vi "Read Current Paths.vi"(11 "PathControl in":refnum<class "PathControl.lvclass">) -> (2 "Current Paths":T1(array[cluster]), 3 "PathControl out":refnum<class "PathControl.lvclass">)   [LabVIEW 2020, in "PathControl.lvclass"]
uses:
  PathControl.lvclass
  PathControl.lvclass/PathControl.ctl
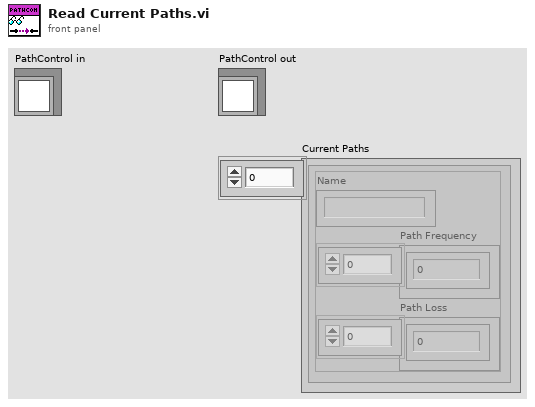
[diagram p1: front panel]
types:
  T1 = cluster{"Name":string, "Path Frequency":dbl[], "Path Loss":dbl[]}[]
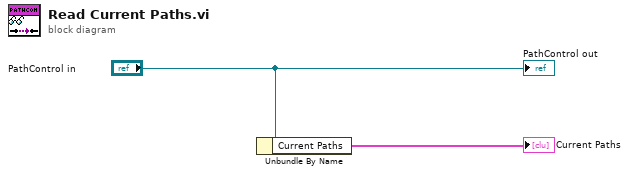
[diagram p0: block diagram]
diagram:
  n1 = Unbundle By Name("PathControl in") -> ("Current Paths"=→"Current Paths":T1)
  "PathControl out" <- "PathControl in"
